vi "Get Attachment Details.vi"(6 "Authorization":T2[](array[typedef]), 8 "error in (no error)":errorcluster, 11 "Attachment GID":string) -> (0 "error out":errorcluster, 2 "download url":string, 3 "data":T1)   [LabVIEW 2016]
uses:
  <vilib>/addons/_JKI.lib/REST Client/classes/REST Client/HTTP Header.ctl
  <vilib>/addons/_JKI.lib/REST Client/classes/REST Client/REST Client.lvclass
  <vilib>/addons/_JKI.lib/Serialization/JSON/JKI JSON Serialization.lvlib
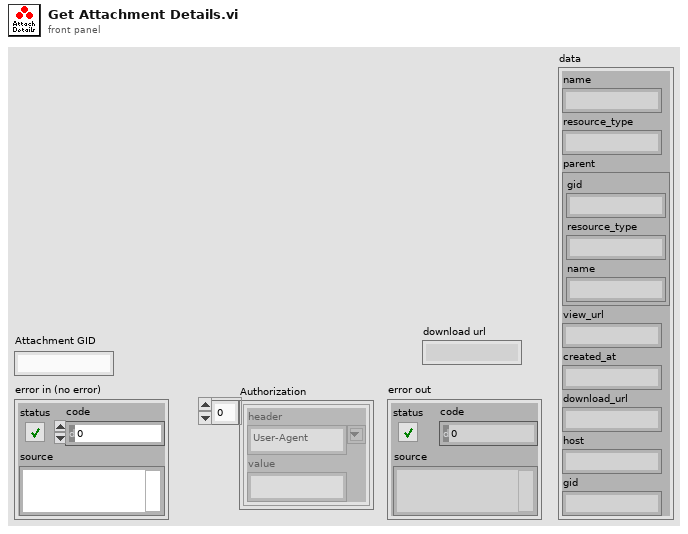
[diagram p1: front panel]
types:
  T1 = cluster{"name":string, "resource_type":string, "parent":cluster{"gid":string, "resource_type":string, "name":string}, "view_url":string, "created_at":string, "download_url":string, "host":string, "gid":string}
  T2 = typedef "REST Client.lvlib/REST Client.lvclass/HTTP Header.ctl" = cluster{"header":string, "value":string}
  T3 = cluster{"data":cluster{"name":string, "resource_type":string, "parent":cluster{"gid":string, "resource_type":string, "name":string}, "view_url":string, "created_at":string, "download_url":string, "host":string, "gid":string}}
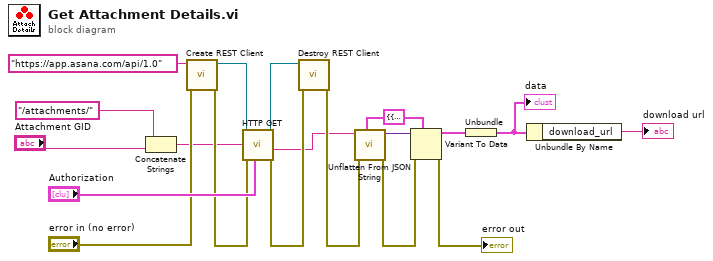
[diagram p0: block diagram]
diagram:
  w4 = T3 {"data"={"name"="", "resource_type"="", "parent"={"gid"="", "resource_type"="", "name"=""}, "view_url"="", "created_at"="", "download_url"="", "host"="", "gid"=""}}
  n1 = Concatenate Strings("/attachments/", "Attachment GID") -> (w11:string)
  n2 = call <vilib>:"Create REST Client.vi"("error in (no error)"="error in (no error)", "Base URL"="https://app.asana.com/api/1.0") -> ("error out"=w14:errorcluster, "REST Client out"=w19:refnum<class "REST Client.lvclass">)  [unwired: 8 in]
  n3 = call-dynamic "HTTP GET.vi"("request specific headers"="Authorization", "error in (no error)"=w14, "Path"=w11, "REST Client in"=w19) -> ("error out"=w10:errorcluster, "Response body"=w8:string, "REST Client out"=w18:refnum<class "REST Client.lvclass">)  [unwired: 2 in, 3 out]
  n4 = call-dynamic "Destroy REST Client.vi"("error in (no error)"=w10, "REST Client in"=w18) -> ("error out"=w9:errorcluster)  [unwired: 9 in]
  n5 = call <vilib>:"Unflatten From JSON String.vi"("Type and Defaults"=w4, "error in (no error)"=w9, "JSON String"=w8) -> ("error out"=w7:errorcluster, "Variant"=w5:variant)  [unwired: 7 in]
  n6 = Variant To Data(error in=w7, type=w4, Variant=w5) -> (data=w3:T3, error out=→"error out":errorcluster)
  n7 = Unbundle(w3) -> ("data"=w2:T1)
  "data" <- w2
  n8 = Unbundle By Name(w2) -> ("download_url"=→"download url":string)
